vi "Testing02.vi"() -> ()   [LabVIEW 2012]
uses:
  <vilib>/Utility/inputDevices.llb/joystickAcquire.vi
  Logging VIs/Update VIs/Logging Update - Numeric Array.vi
  femtoRoboLib.lvlib
panel:
  out "Playback Time":u32
  in  "Replay":bool
  out "Waveform Graph":waveform(dbl)[](graph)
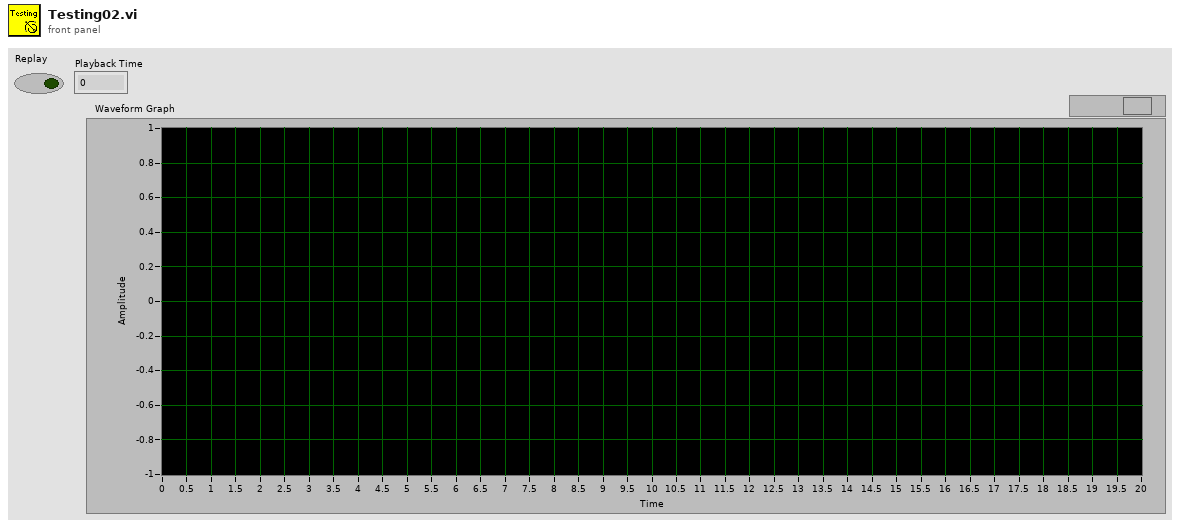
[diagram p1: front panel]
types:
  T1 = typedef "femtoRoboLib.lvlib/LoggingDevRef.ctl" = cluster{"DevStatus":errorcluster, "refnum":refnum<file>, "Path":path, "Start Time":u32}
  T2 = cluster{"X axis":i32, "Y axis":i32, "Z axis":i32, "X axis rotation":i32, "Y axis rotation":i32, "Z axis rotation":i32, "U axis":i32, "V axis":i32}
  T3 = typedef "femtoRoboLib.lvlib/Log Entry - Full Block.ctl" = cluster{"Entries":T4[], "Time":u32}
  T4 = typedef "femtoRoboLib.lvlib/Log Entry.ctl" = cluster{"Name":string, "Type":T5, "Value":T6}
  T5 = typedef "femtoRoboLib.lvlib/Log Value Type.ctl" = enum16{"Boolean", "Numeric", "String", "Boolean Array", "Numeric Array", "String Array"}
  T6 = typedef "femtoRoboLib.lvlib/Log Value Cluster.ctl" = cluster{"Boolean Array":bool[], "Boolean":bool, "Numeric Array":dbl[], "Numeric":dbl, "String Array":string[], "String":string}
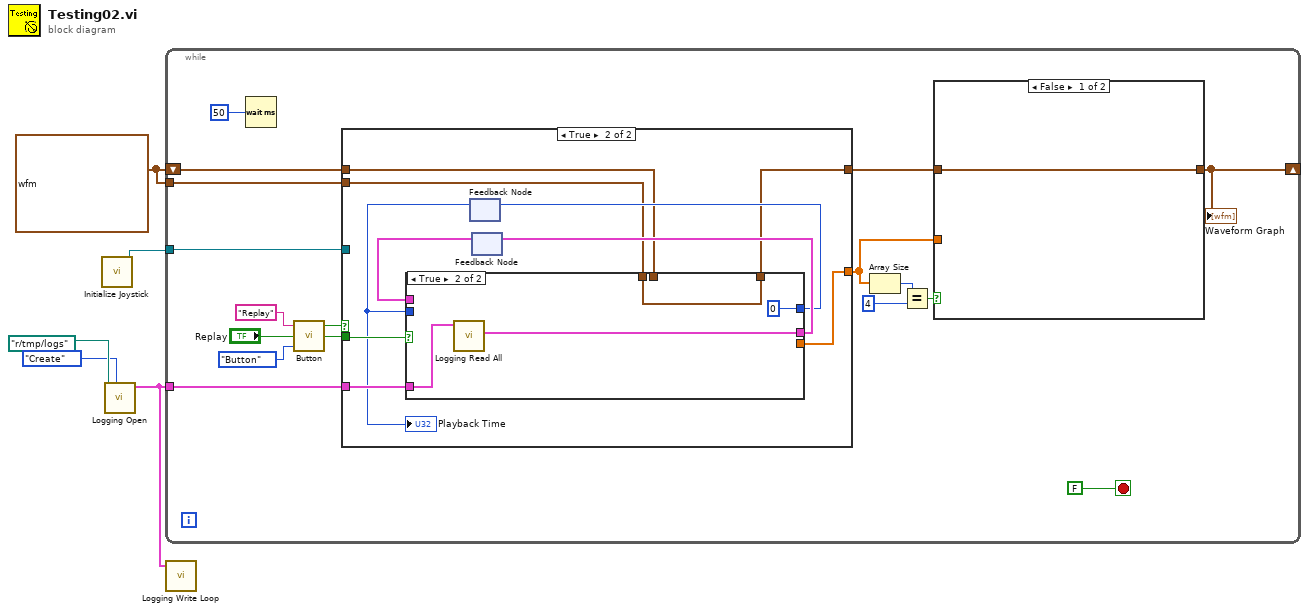
[diagram p0: block diagram]
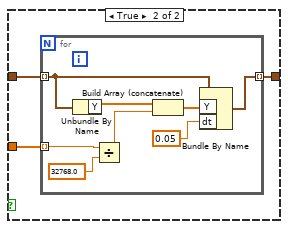
[diagram p2: hidden frame]
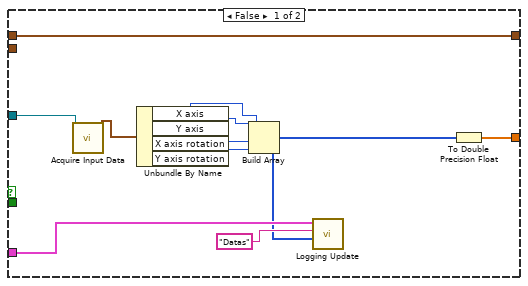
[diagram p3: hidden frame]
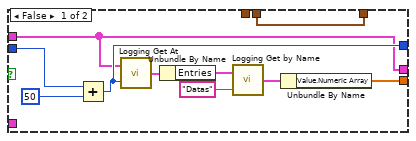
[diagram p4: hidden frame]
diagram:
  w1 = waveform(dbl)[] [{"t0"=timestamp(0 s since 1904-01-01), "dt"=1.0, "Y"=[]}, {"t0"=timestamp(0 s since 1904-01-01), "dt"=1.0, "Y"=[]}, {"t0"=timestamp(0 s since 1904-01-01), "dt"=1.0, "Y"=[]}, {"t0"=timestamp(0 s since 1904-01-01), "dt"=1.0, "Y"=[]}] ("Array")
  n1 = call <vilib>:"Initialize Joystick.vi"() -> ("device ID"=w5:refnum<k1>)  [unwired: 10 in, 1 out]
  n2 = call "Logging Open.vi"("Mode"=enum16{"Create", "Open"}."Create", "base path"=path "r:/tmp/logs" ("palette path")) -> ("LoggingDevRef"=w2:T1)  [unwired: 7 in, 1 out]
  n3 = while {
    tunnel: w5 -> [w22]
    shift-right: [w21] -> _
    shift-left: w1 -> [w12]
    tunnel: w2 -> [w18]
    tunnel: w1 -> [w10]
    stop <- FALSE stop-if-true
    n4 = Wait (ms)(milliseconds to wait=u32 50) -> ()  [unwired: 1 out]
    n5 = call "Button.vi"("Set Mode"=enum16{"Noop", "Button", "Switch"}."Button", "In"="Replay", "Name"="Replay") -> ("Leading"=w13:bool, "Out"=w14:bool)  [unwired: 1 out]
    n6 = case shown="True" w14 {
      tunnel: w22 -> [w45 _]
      tunnel: [w36 w50] -> w9
      tunnel: w18 -> [w39 w54]
      tunnel: w13 -> [_ w55]
      tunnel: w12 -> [w35 w49]
      tunnel: [w35 w48] -> w11
      tunnel: w10 -> [_ w47]
      frame False {
        n7 = call-poly <vilib>:"Acquire Input Data.vi"("device ID"=w45) -> ("axis info"=w44:T2)  [unwired: 14 in, 4 out]
        n8 = Unbundle By Name(w44) -> ("X axis"=w42:i32, "Y axis"=w43:i32, "X axis rotation"=w41:i32, "Y axis rotation"=w40:i32)
        n9 = Build Array(w42, w43, w41, w40) -> (w37:i32[])
        n10 = call-poly "Logging Update.vi"("Value"=w37, "Name"="Datas", "LoggingDevRef"=w39) -> ()  [unwired: 3 in, 2 out]
        n11 = To Double Precision Float(number=w37) -> (double precision float=w36:dbl[])
      }
      frame True {
        n12 = feedback #1() -> (w46:u32)  [unwired: 1 in]
        "Playback Time" <- w46
        n13 = feedback #2() -> (w52:T3[])  [unwired: 1 in]
        n14 = case shown="True" w55 {
          tunnel: w54 -> [_ w69]
          tunnel: w52 -> [w58 _]
          tunnel: [w58 w68] -> w53
          tunnel: w46 -> [w64 _]
          tunnel: [w63 u32 0] -> w51
          tunnel: [w57 _] -> w50
          tunnel: w49 -> [w56 _]
          tunnel: [w56 w66] -> w48
          tunnel: w47 -> [_ w66]
          frame False {
            n15 = Add(x=w64, y=u32 50) -> (x+y=w63:u32)
            n16 = call "Logging Get At.vi"("Time (ms)"=w63, "Log Input"=w58) -> ("Output"=w62:T3)
            n17 = Unbundle By Name(w62) -> ("Entries"=w61:T4[])
            n18 = call "Logging Get by Name.vi"("Name"="Datas", "Entries"=w61) -> ("Entry"=w59:T4)
            n19 = Unbundle By Name(w59) -> ("Value.Numeric Array"=w57:dbl[])
          }
          frame True {
            n20 = call "Logging Read All.vi"("LoggingDevRef"=w69) -> ("Log"=w68:T3[])  [unwired: 4 in, 2 out]
          }
        }
        n21 = feedback-in #1(w51) -> ()
        n22 = feedback-in #2(w53) -> ()
      }
    }
    n23 = Array Size(array=w9) -> (size(s)=w8:i32)
    n24 = Equal?(x=w8, y=4) -> (x = y?=w7:bool)
    n25 = case shown="False" w7 {
      tunnel: w9 -> [_ w26]
      tunnel: [w23 w25] -> w21
      tunnel: w11 -> [w23 w24]
      frame False {
      }
      frame True {
        n26 = for {
          tunnel: w24 -> [w29] mode=indexing
          tunnel: w26 -> [w27] mode=indexing
          tunnel: [w28] -> w25 mode=indexing
          n27 = Unbundle By Name(w29) -> ("Y"=w33:dbl[])
          n28 = Divide(x=w27, y=32768.0) -> (x/y=w32:dbl)
          n29 = Build Array (concatenate)(w33, w32) -> (w31:dbl[])
          n30 = Bundle By Name(cluster=w29, "Y"=w31, "dt"=0.05) -> (w28:waveform(dbl))
        }
      }
    }
    "Waveform Graph" <- w21
  }
  n31 = call "Logging Write Loop.vi"("LoggingDevRef"=w2) -> ()  [unwired: 5 in]
